vi "PicoScope2000AdvancedTriggerSettings.vi"(0 "handle in":i16=16384, 2 "Pulse Width Qualifier Conditions":T4 {"Condition Logic" items=["AND", "OR", "XOR"]}, 3 "Pulse Width Qualifier Settings":T3={"Direction"=2, "Lower Limit"=0, "Upper Limit"=0, "Pulse Width Type"=0} {"Pulse Width Type" items=["None", "Less Than", "Greater Than", "In Range", "Out of Range"]; "Direction" items=["Rising"=2, "Falling"=3]}, 5 "error in":errorcluster, 6 "Trigger Conditions":T1 {"PWQ" items=["Don't Care", "True", "False"]; "Ext" items=["Don't Care", "True", "False"]; "Channel D" items=["Don't Care", "True", "False"]; "Channel C" items=["Don't Care", "True", "False"]; "Channel B" items=["Don't Care", "True", "False"]; "Channel A" items=["Don't Care", "True", "False"]; "Condition Logic" items=["AND", "OR", "XOR"]}, 7 "Auto Trigger (ms)":i32=1000, 8 "Channel A Trigger Properties":T2={"thresholdUpper"=0, "thresholdHysteresis"=0, "thresholdLower"=0, "Threshold Mode"=0, "Direction"=2, "Available"=FALSE} {"Direction" items=["Above / Inside", "Below / Outside", "Rising / Enter", "Falling / Exit", "Rising or Falling / Enter or Exit", "Above Lower", "Below Lower", "Rising Lower", "Falling Lower", "Positive Runt", "Negative Runt"]; "Threshold Mode" items=["Level", "Window"]}, 9 "Trigger Delay":u32, 10 "Channel B Trigger Properties":T2={"thresholdUpper"=0, "thresholdHysteresis"=0, "thresholdLower"=0, "Threshold Mode"=0, "Direction"=2, "Available"=FALSE} {"Direction" items=["Above / Inside", "Below / Outside", "Rising / Enter", "Falling / Exit", "Rising or Falling / Enter or Exit", "Above Lower", "Below Lower", "Rising Lower", "Falling Lower", "Positive Runt", "Negative Runt"]; "Threshold Mode" items=["Level", "Window"]}, 11 "preTriggerDelay":sgl, 12 "Ext. Trigger Properties":T2={"thresholdUpper"=0, "thresholdHysteresis"=0, "thresholdLower"=0, "Threshold Mode"=0, "Direction"=2, "Available"=FALSE} {"Direction" items=["Above / Inside", "Below / Outside", "Rising / Enter", "Falling / Exit", "Rising or Falling / Enter or Exit", "Above Lower", "Below Lower", "Rising Lower", "Falling Lower", "Positive Runt", "Negative Runt"]; "Threshold Mode" items=["Level", "Window"]}) -> (14 "handle out":i16=16384, 19 "error out":errorcluster)   [LabVIEW 2010]
doc: "This VI is an interface for the advanced trigger features of the oscilloscope (a simple trigger can be set using PicoScope2000Settings.vi, in which case it is not necessary to use this VI)."
uses:
  ps2000.dll
panel:
  in  "Channel D Trigger Properties":T2={"thresholdUpper"=0, "thresholdHysteresis"=0, "thresholdLower"=0, "Threshold Mode"=0, "Direction"=2, "Available"=FALSE} {"Direction" items=["Above / Inside", "Below / Outside", "Rising / Enter", "Falling / Exit", "Rising or Falling / Enter or Exit", "Above Lower", "Below Lower", "Rising Lower", "Falling Lower", "Positive Runt", "Negative Runt"]; "Threshold Mode" items=["Level", "Window"]}
  in  "Channel C Trigger Properties":T2={"thresholdUpper"=0, "thresholdHysteresis"=0, "thresholdLower"=0, "Threshold Mode"=0, "Direction"=2, "Available"=FALSE} {"Direction" items=["Above / Inside", "Below / Outside", "Rising / Enter", "Falling / Exit", "Rising or Falling / Enter or Exit", "Above Lower", "Below Lower", "Rising Lower", "Falling Lower", "Positive Runt", "Negative Runt"]; "Threshold Mode" items=["Level", "Window"]}
  # "For Condition Logic Suggested settings;\nFor AND, XOR logic-(parallel triggers)\nUse level-type triggers (Level or Inside/outside Window Triggers)\n\nFor OR logic- (single channel)\nUse edge types (e.g. rising, falling, entering window)"
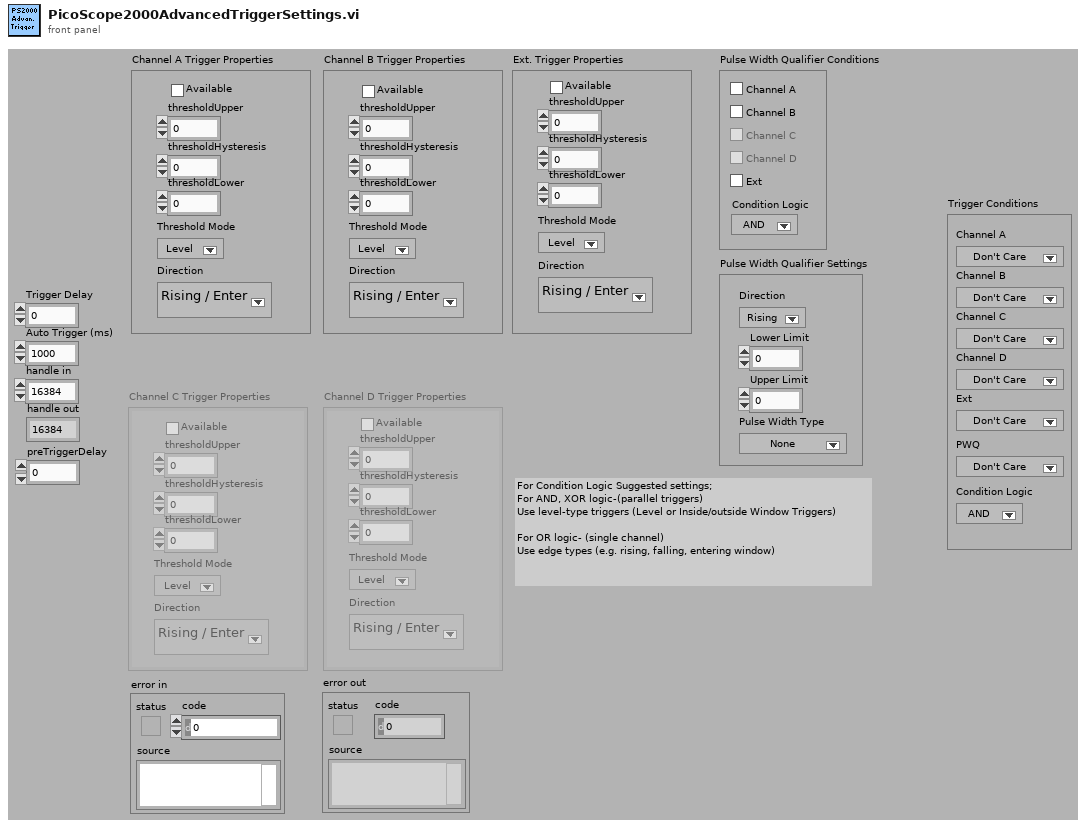
[diagram p1: front panel]
types:
  T1 = cluster{"Channel A":u16, "Channel B":u16, "Channel C":u16, "Channel D":u16, "Ext":u16, "PWQ":u16, "Condition Logic":u16}
  T2 = cluster{"thresholdUpper":i16, "thresholdHysteresis":u16, "thresholdLower":i16, "Threshold Mode":i32, "Direction":i32, "Available":bool}
  T3 = cluster{"Direction":u32, "Lower Limit":u32, "Upper Limit":u32, "Pulse Width Type":u32}
  T4 = cluster{"Channel A":bool, "Channel B":bool, "Channel C":bool, "Channel D":bool, "Condition Logic":u16, "Ext":bool}
  T5 = cluster{"thresholdUpper":i16, "thresholdHysteresis":u16, "thresholdLower":i16, "Threshold Mode":i32, "Direction":i32, "Available":bool}[]
  T6 = cluster{"[0]":u32, "[1]":u32, "[2]":u32, "[3]":u32, "[4]":u32, "[5]":u32, "[6]":u32, "[7]":u32, "[8]":u32}
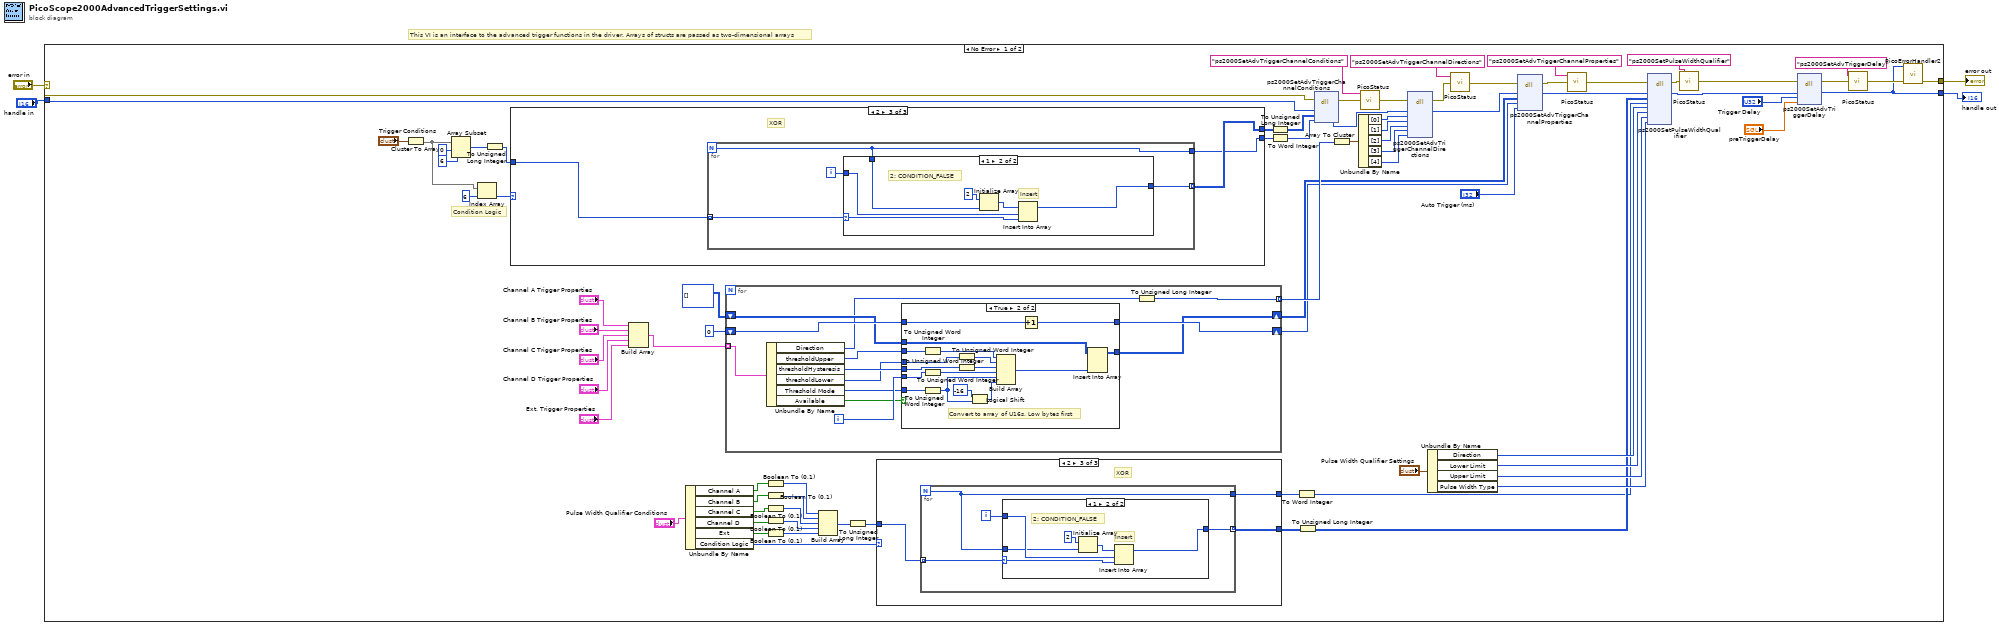
[diagram p0: block diagram]
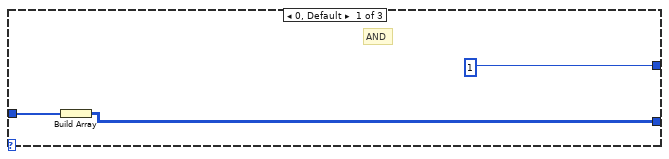
[diagram p2: hidden frame]
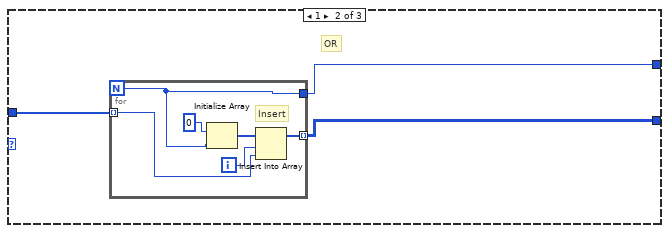
[diagram p3: hidden frame]
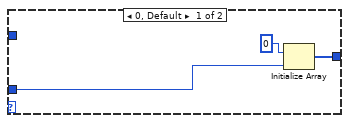
[diagram p4: hidden frame]
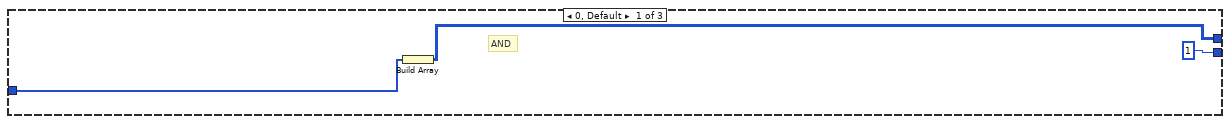
[diagram p6: hidden frame]
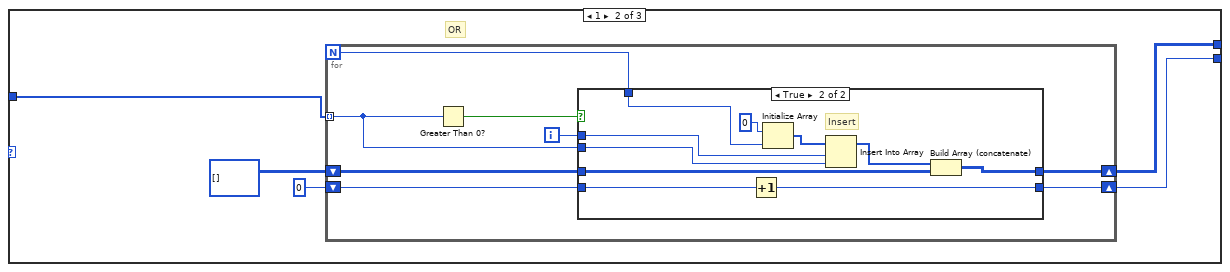
[diagram p7: hidden frame]
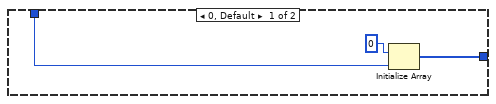
[diagram p9: hidden frame]
diagram:
  # "This VI is an interface to the advanced trigger functions in the driver. Arrays of structs are passed as two-dimensional arrays"
  n1 = case shown="No Error" "error in" {
    selector: "error in" -> [w57 w187]
    tunnel: "handle in" -> [w60 w188]
    tunnel: [w34 w188] -> w2
    tunnel: [w35 w187] -> w1
    frame No Error {
      # "Condition Logic"
      n2 = Cluster To Array(cluster="Trigger Conditions") -> (array=w5:u16[])
      n3 = Array Subset(array=w5, index=0, length=6) -> (w8:u16[])
      n4 = Index Array(array=w5, index=6) -> (element=w6:u16)
      n5 = To Unsigned Long Integer(number=w8) -> (unsigned 32bit integer=w27:u32[])
      n6 = case shown="2" w6 {
        tunnel: [w145 w150 w173] -> w41
        tunnel: [i16 1 w146 w171] -> w26
        tunnel: w27 -> [w143 w147 w172]
        frame 0, Default {
          # "AND"
          n7 = Build Array(w143) -> (w145:u32[][])
        }
        frame 1 {
          # "OR"
          n8 = for {
            N -> [w151]
            tunnel: w147 -> [w155] mode=indexing
            shift-right: [w154] -> w150
            shift-left: u32[][] [] -> [w158]
            shift-right: [w152] -> w146
            shift-left: 0 -> [w153]
            i -> [w157]
            n9 = Greater Than 0?(x=w155) -> (x > 0?=w156:bool)
            n10 = case shown="True" w156 {
              tunnel: w158 -> [w160 w164]
              tunnel: w157 -> [_ w168]
              tunnel: w155 -> [_ w167]
              tunnel: [w160 w166] -> w154
              tunnel: w153 -> [w159 w163]
              tunnel: [w159 w162] -> w152
              tunnel: w151 -> [_ w161]
              frame False {
              }
              frame True {
                # "Insert"
                n11 = Increment(x=w163) -> (x+1=w162:i32)
                n12 = Initialize Array(u32 0 ("element"), w161) -> (w169:u32[])
                n13 = Insert Into Array(array=w169, index=w168, new element=w167) -> (w165:u32[])
                n14 = Build Array (concatenate)(w165, w164) -> (w166:u32[][])
              }
            }
          }
        }
        frame 2 {
          # "XOR"
          n15 = for {
            N -> [w174]
            tunnel: w172 -> [w175] mode=indexing
            tunnel: [w177] -> w173 mode=indexing
            tunnel: [w174] -> w171
            i -> [w176]
            n16 = case shown="1" w175 {
              selector: w175 -> [_ w183]
              tunnel: [w179 w184] -> w177
              tunnel: w176 -> [_ w182]
              tunnel: w174 -> [w178 w181]
              frame 0, Default {
                n17 = Initialize Array(0 ("element"), w178) -> (w179:i32[])
              }
              frame 1 {
                # "2: CONDITION_FALSE"
                # "Insert"
                n18 = Initialize Array(u32 2 ("element"), w181) -> (w185:u32[])
                n19 = Insert Into Array(array=w185, index=w182, new element=w183) -> (w184:u32[])
              }
            }
          }
        }
      }
      n20 = Build Array("Channel A Trigger Properties", "Channel B Trigger Properties", "Channel C Trigger Properties", "Channel D Trigger Properties", "Ext. Trigger Properties") -> (w79:T5)
      n21 = Unbundle By Name("Pulse Width Qualifier Conditions") -> ("Channel A"=w15:bool, "Channel B"=w16:bool, "Channel C"=w17:bool, "Channel D"=w18:bool, "Ext"=w19:bool, "Condition Logic"=w14:u16)
      n22 = for {
        tunnel: w79 -> [w120] mode=indexing
        tunnel: [w113] -> w78 mode=indexing
        shift-right: [w118] -> w47
        shift-left: i16 0 -> [w117]
        shift-right: [w115] -> w45
        shift-left: u16[][] [] -> [w116]
        i -> [w119]
        n23 = Unbundle By Name(w120) -> ("Direction"=w114:i32, "thresholdUpper"=w123:i16, "thresholdHysteresis"=w122:u16, "thresholdLower"=w121:i16, "Threshold Mode"=w111:i32, "Available"=w112:bool)
        n24 = case shown="True" w112 {
          tunnel: w123 -> [_ w137]
          tunnel: w122 -> [_ w136]
          tunnel: w121 -> [_ w135]
          tunnel: w111 -> [_ w127]
          tunnel: w119 -> [_ w134]
          tunnel: [w125 w142] -> w118
          tunnel: w117 -> [w125 w141]
          tunnel: [w124 w139] -> w115
          tunnel: w116 -> [w124 w138]
          frame False {
          }
          frame True {
            # "Convert to array of U16s, Low bytes first"
            n25 = To Unsigned Word Integer(number=w137) -> (unsigned 16bit integer=w133:u16)
            n26 = To Unsigned Word Integer(number=w134) -> (unsigned 16bit integer=w130:u16)
            n27 = To Unsigned Word Integer(number=w127) -> (unsigned 16bit integer=w126:u16)
            n28 = To Unsigned Word Integer(number=w135) -> (unsigned 16bit integer=w132:u16)
            n29 = To Unsigned Word Integer(number=w136) -> (unsigned 16bit integer=w131:u16)
            n30 = Logical Shift(y=i16 -16, x=w126) -> (x << y=w128:u16)
            n31 = Build Array(w133, w132, w131, w130, w126, w128) -> (w140:u16[])
            n32 = Increment(x=w141) -> (x+1=w142:i16)
            n33 = Insert Into Array(array=w138, new element=w140) -> (w139:u16[][])  [unwired: 2 in]
          }
        }
        n34 = To Unsigned Long Integer(number=w114) -> (unsigned 32bit integer=w113:u32)
      }
      n35 = Boolean To (0,1)(Boolean=w15) -> (0, 1=w24:i16)
      n36 = Boolean To (0,1)(Boolean=w16) -> (0, 1=w23:i16)
      n37 = Boolean To (0,1)(Boolean=w17) -> (0, 1=w22:i16)
      n38 = Boolean To (0,1)(Boolean=w18) -> (0, 1=w21:i16)
      n39 = Boolean To (0,1)(Boolean=w19) -> (0, 1=w20:i16)
      n40 = Build Array(w24, w23, w22, w21, w20) -> (w13:i16[])
      n41 = To Unsigned Long Integer(number=w13) -> (unsigned 32bit integer=w12:u32[])
      n42 = case shown="2" w14 {
        tunnel: [w85 w88 w97] -> w40
        tunnel: [i16 1 w87 w96] -> w28
        tunnel: w12 -> [w83 w86 w95]
        frame 0, Default {
          # "AND"
          n43 = Build Array(w83) -> (w85:u32[][])
        }
        frame 1 {
          # "OR"
          n44 = for {
            N -> [w89]
            tunnel: w86 -> [w91] mode=indexing
            tunnel: [w90] -> w88 mode=indexing
            tunnel: [w89] -> w87
            i -> [w92]
            # "Insert"
            n45 = Initialize Array(u32 0 ("element"), w89) -> (w93:u32[])
            n46 = Insert Into Array(array=w93, index=w92, new element=w91) -> (w90:u32[])
          }
        }
        frame 2 {
          # "XOR"
          n47 = for {
            N -> [w98]
            tunnel: w95 -> [w101] mode=indexing
            tunnel: [w99] -> w97 mode=indexing
            tunnel: [w98] -> w96
            i -> [w100]
            n48 = case shown="1" w101 {
              selector: w101 -> [_ w107]
              tunnel: [w103 w108] -> w99
              tunnel: w100 -> [_ w106]
              tunnel: w98 -> [w102 w105]
              frame 0, Default {
                n49 = Initialize Array(u32 0 ("element"), w102) -> (w103:u32[])
              }
              frame 1 {
                # "2: CONDITION_FALSE"
                # "Insert"
                n50 = Initialize Array(u32 2 ("element"), w105) -> (w109:u32[])
                n51 = Insert Into Array(array=w109, index=w106, new element=w107) -> (w108:u32[])
              }
            }
          }
        }
      }
      n52 = To Unsigned Long Integer(number=w41) -> (unsigned 32bit integer=w42:u32[][])
      n53 = To Word Integer(number=w26) -> (16bit integer=w25:i16)
      n54 = To Word Integer(number=w28) -> (16bit integer=w29:i16)
      n55 = To Unsigned Long Integer(number=w40) -> (unsigned 32bit integer=w39:u32[][])
      n56 = dll-call lib="ps2000.dll" fn="ps2000SetAdvTriggerChannelConditions" ("ps3000.dll:_ps3000_open_unit@0")(error in=w57, "handle"=w60, "conditions"=w42, "nConditions"=w25) -> (error out=w59:errorcluster, "handle"=w38:i16)  [unwired: 5 in, 1 out]
      n57 = Array To Cluster(array=w78) -> (cluster=w77:T6)
      n58 = Unbundle By Name(w77) -> ("[0]"=w76:u32, "[1]"=w75:u32, "[2]"=w74:u32, "[3]"=w73:u32, "[4]"=w72:u32)
      n59 = call "PicoStatus.vi"("error in"=w59, "source"="ps2000SetAdvTriggerChannelConditions") -> ("error out"=w37:errorcluster)  [unwired: 1 in]
      n60 = dll-call lib="ps2000.dll" fn="ps2000SetAdvTriggerChannelDirections" ("ps3000.dll:_ps3000_open_unit@0")(error in=w37, "handle"=w38, "channelA"=w76, "channelB"=w75, "channelC"=w74, "channelD"=w73, "ext"=w72) -> (error out=w56:errorcluster, "handle"=w82:i16)  [unwired: 8 in, 1 out]
      n61 = Unbundle By Name("Pulse Width Qualifier Settings") -> ("Direction"=w68:u32, "Lower Limit"=w67:u32, "Upper Limit"=w66:u32, "Pulse Width Type"=w65:u32)
      n62 = call "PicoStatus.vi"("error in"=w56, "source"="ps2000SetAdvTriggerChannelDirections") -> ("error out"=w53:errorcluster)  [unwired: 1 in]
      n63 = dll-call lib="ps2000.dll" fn="ps2000SetAdvTriggerChannelProperties" ("ps3000.dll:_ps3000_open_unit@0")(error in=w53, "handle"=w82, "channelProperties"=w45, "nChannelProperties"=w47, "autoTriggerMilliseconds"="Auto Trigger (ms)") -> (error out=w55:errorcluster, "handle"=w81:i16)  [unwired: 6 in, 1 out]
      n64 = call "PicoStatus.vi"("error in"=w55, "source"="ps2000SetAdvTriggerChannelProperties") -> ("error out"=w52:errorcluster)  [unwired: 1 in]
      n65 = dll-call lib="ps2000.dll" fn="ps2000SetPulseWidthQualifier" ("ps3000.dll:_ps3000_open_unit@0")(error in=w52, "handle"=w81, "conditions"=w39, "nConditions"=w29, "direction"=w68, "lower"=w67, "upper"=w66, "type"=w65) -> (error out=w54:errorcluster, "handle"=w43:i16)  [unwired: 9 in, 1 out]
      n66 = call "PicoStatus.vi"("error in"=w54, "source"="ps2000SetPulseWidthQualifier") -> ("error out"=w44:errorcluster)  [unwired: 1 in]
      n67 = dll-call lib="ps2000.dll" fn="ps2000SetAdvTriggerDelay" ("ps3000.dll:_ps3000_open_unit@0")(error in=w44, "handle"=w43, "delay"="Trigger Delay", "preTriggerDelay"="preTriggerDelay") -> (error out=w33:errorcluster, "handle"=w34:i16)  [unwired: 5 in, 1 out]
      n68 = call "PicoStatus.vi"("error in"=w33, "source"="ps2000SetAdvTriggerDelay") -> ("error out"=w36:errorcluster)  [unwired: 1 in]
      n69 = call "PicoErrorHandler2.vi"("error in (no error)"=w36, "handle In"=w34) -> ("error out"=w35:errorcluster)  [unwired: 9 in]
    }
    frame Error {
    }
  }
  "handle out" <- w2
  "error out" <- w1
